vi "Complex FIR Filter (real signal).vi"(2 "init/cont (init:F)":bool, 3 "FIR Coefficients":cdb[](array[numeric]), 5 "X":dbl[](array[numeric])) -> (0 "error":i32, 1 "Filtered X":cdb[](array[numeric]))   [LabVIEW 2014, in "NI_AALBase.lvlib"]
uses:
  NI_AALBase.lvlib
  lvanlys.dll
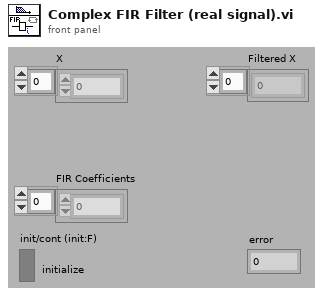
[diagram p1: front panel]
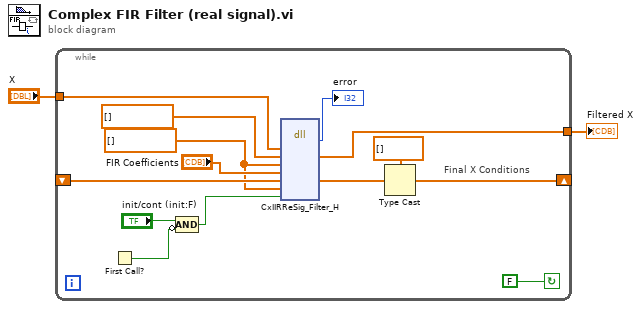
[diagram p0: block diagram]
diagram:
  n1 = while {
    shift-left: _ -> [w10]
    shift-right: [w16] -> _
    tunnel: "X" -> [w13]
    tunnel: [w7] -> w1
    stop <- FALSE continue-if-true
    w3 = cdb[] [] ("Reverse Coefficients")
    # "Final X Conditions"
    n2 = First Call?() -> (First Call?: T/F=w12:bool)
    n3 = Compound Arithmetic op=AND("init/cont (init:F)", invert w12) -> (w11:bool)
    n4 = dll-call lib="C:/Program Files (x86)/National Instruments/LabVIEW 2014/resource/lvanlys.*" fn="CxIIRReSig_Filter_H"("xH"=w13, "Y"=cdb[] [], "Reverse Coefficients"=w3, "FIR Coefficients"="FIR Coefficients", "x1H"=w10, "Reverse Coefficients"=w3, w11) -> (→"error":i32, "Y"=w7:cdb[], "x1H"=w9:dbl[])  [unwired: 8 in, 2 out]
    n5 = Type Cast(type=dbl[] [], x=w9) -> (*(type *) &x=w16:dbl[])
  }
  "Filtered X" <- w1
